vi "Update Value.vi"(6 "Timestamp (Now)":dbl, 8 "error in (no error)":errorcluster, 9 "Raw Value":dbl, 10 "Value":dbl, 11 "Channel in":refnum<class "Channel DBL.lvclass">) -> (0 "error out":errorcluster, 3 "Channel out":refnum<class "Channel DBL.lvclass">)   [LabVIEW 2020, in "Vecto.lvlib" / "Channel DBL.lvclass"]
uses:
  Channel DBL.lvclass
  Channel DBL.lvclass/Channel DBL.ctl
  Group DBL/Group DBL.lvclass
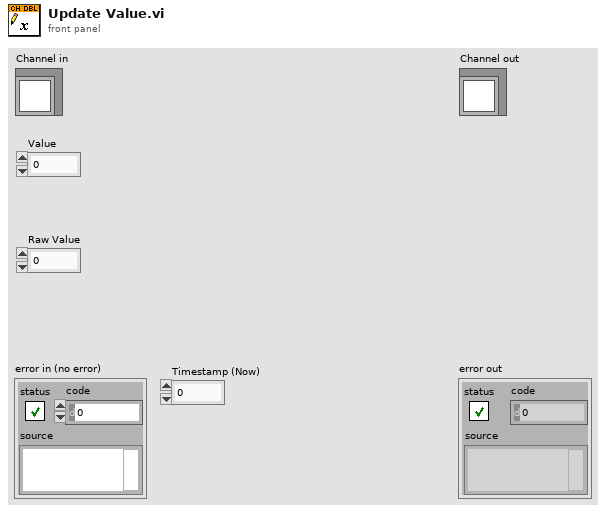
[diagram p1: front panel]
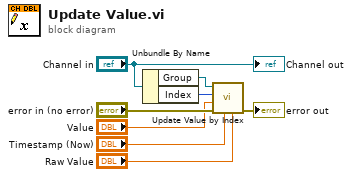
[diagram p0: block diagram]
diagram:
  n1 = Unbundle By Name("Channel in") -> ("Group"=w6:refnum<class "Group DBL.lvclass">, "Index"=w5:i32)
  n2 = call "Update Value by Index.vi"("Raw"="Raw Value", "Timestamp (Now)"="Timestamp (Now)", "error in (no error)"="error in (no error)", "Scaled"="Value", "Index"=w5, "Group in"=w6) -> ("error out"=→"error out":errorcluster)  [unwired: 4 in, 1 out]
  "Channel out" <- "Channel in"
